vi "Get_STL.vi"(8 "error in":errorcluster, 11 "Device In":T1) -> (0 "error out":errorcluster, 1 "stl text":string, 2 "Comm":T2, 3 "Device Out":T1)   [LabVIEW 2019]
uses:
  <userlib>/IoT Devices/_subVIs/HTTPComm.ctl
  <userlib>/Onshape/_SubVI/Cluster.ctl
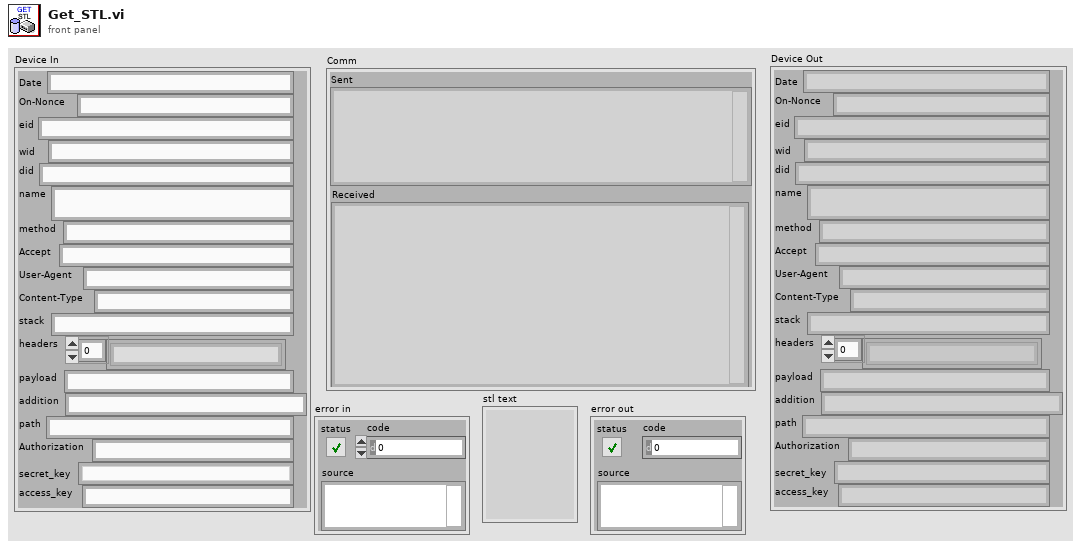
[diagram p1: front panel]
types:
  T1 = typedef "Cluster.ctl" = cluster{"Date":string, "On-Nonce":string, "eid":string, "wid":string, "did":string, "name":string, "method":string, "Accept":string, "User-Agent":string, "Content-Type":string, "stack":string, "headers":string[], "payload":string, "addition":string, "path":string, "Authorization":string, "secret_key":string, "access_key":string}
  T2 = typedef "HTTPComm.ctl" = cluster{"url":string, "sent headers":string, "sent body":string, "headers":string, "body":string, "Sent":string, "Received":string}
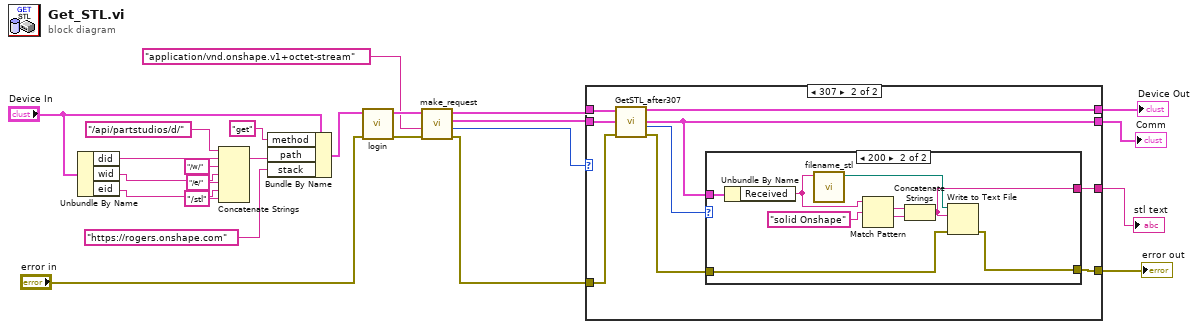
[diagram p0: block diagram]
diagram:
  n1 = Unbundle By Name("Device In") -> ("did"=w17:string, "wid"=w13:string, "eid"=w11:string)
  n2 = Concatenate Strings("/api/partstudios/d/" ("payload"), w17, "/w/" ("string"), w13, "/e/" ("string"), w11, "/stl" ("string")) -> (w22:string)
  n3 = Bundle By Name(cluster="Device In", "method"="get" ("Method"), "path"=w22, "stack"="https://rogers.onshape.com" ("stacks")) -> (w19:T1)
  n4 = call <userlib>:"login.vi"("error in"="error in", "Device In"=w19) -> ("error out"=w20:errorcluster, "Device Out"=w18:T1)  [unwired: 8 in]
  n5 = call <userlib>:"make_request.vi"("Error in"=w20, "Accept"="application/vnd.onshape.v1+octet-stream", "Device In"=w18) -> ("error out"=w7:errorcluster, "error"=w8:i32, "Comm"=w6:T2, "Device Out"=w5:T1)  [unwired: 4 in, 1 out]
  n6 = case shown="307" w8 {
    tunnel: w7 -> [w25 w36]
    tunnel: w6 -> [w26 w35]
    tunnel: w5 -> [w27 w34]
    tunnel: [w27 w33] -> w4
    tunnel: [w26 w32] -> w3
    tunnel: [w25 w29] -> w2
    tunnel: [_ w28] -> w1
    frame 0, Default {
    }
    frame 307 {
      n7 = call <userlib>:"GetSTL_after307.vi"("error in (no error)"=w36, "Comm in"=w35, "Device in"=w34) -> ("error out"=w30:errorcluster, "error"=w31:i32, "Comm out"=w32:T2, "Device Out"=w33:T1)  [unwired: 5 in]
      n8 = case shown="200" w31 {
        tunnel: w32 -> [_ w46]
        tunnel: [w37 w39] -> w29
        tunnel: w30 -> [w37 w40]
        tunnel: [_ w38] -> w28
        frame 0, Default {
        }
        frame 200 {
          n9 = Unbundle By Name(w46) -> ("Received"=w42:string)
          n10 = call <userlib>:"filename_stl.vi"("Received"=w42) -> ("appended path"=w41:path)  [unwired: 10 in]
          n11 = Match Pattern(string=w42, regular expression="solid Onshape") -> (match substring=w44:string, after substring=w43:string)  [unwired: 1 in, 2 out]
          n12 = Concatenate Strings(w44, w43) -> (w38:string)
          n13 = Write to Text File(file (use dialog)=w41, text=w38, error in=w40) -> (error out=w39:errorcluster)  [unwired: 1 in, 2 out]
        }
      }
    }
  }
  "Device Out" <- w4
  "Comm" <- w3
  "error out" <- w2
  "stl text" <- w1
